vi "Populate File Info.vi"(8 "error in":errorcluster, 11 "UI Actor in":refnum<class "UI Actor.lvclass">) -> (0 "error out":errorcluster)   [LabVIEW 2019, in "UI Actor.lvlib" / "UI Actor.lvclass"]
uses:
  UI Actor.lvclass
  UI Actor.lvclass/UI Actor.ctl
  Electronic Datasheet/Electronic Datasheet.lvclass
  Core/File Info/File Info.lvclass
  Controls/File Info.ctl
  UI Actor.lvlib
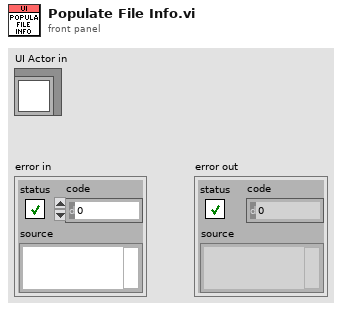
[diagram p1: front panel]
types:
  T1 = typedef "UI Actor.lvlib/File Info.ctl" = cluster{"FileVersion":u8, "FileRevision":u8, "EDSVersion":string, "Description":string, "CreationDate":string, "CreationTime":string, "CreatedBy":string, "ModificationDate":string, "ModificationTime":string, "ModifiedBy":string}
  T2 = map{path, refnum<class "Electronic Datasheet.lvclass">}
  T3 = cluster{"FileName":string, "FileVersion":u8, "FileRevision":u8, "EDSVersion":string, "Description":string, "CreationTime":string, "CreationDate":string, "CreatedBy":string, "ModificationTime":string, "ModificationDate":string, "ModifiedBy":string}
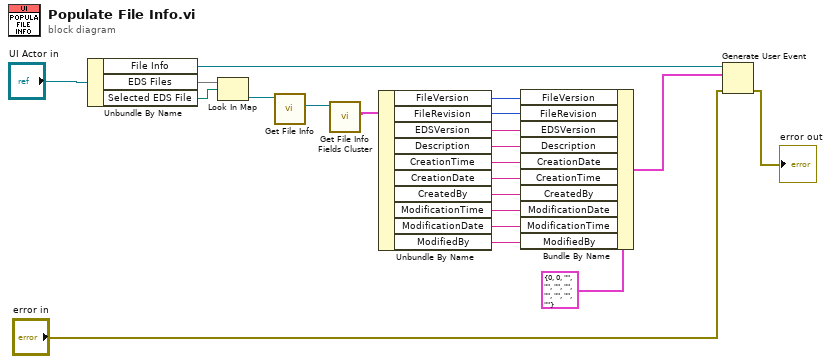
[diagram p0: block diagram]
diagram:
  n1 = Unbundle By Name("UI Actor in") -> ("File Info"=w21:refnum<user-event>, "EDS Files"=w17:T2, "Selected EDS File"=w16:path)
  n2 = Look In Map(map=w17, key=w16) -> (value=w18:refnum<class "Electronic Datasheet.lvclass">)  [unwired: 1 in, 1 out]
  n3 = call "Get File Info.vi"("reference in"=w18) -> ("File Info"=w15:refnum<class "File Info.lvclass">)  [unwired: 9 in, 1 out]
  n4 = call "Get File Info Fields Cluster.vi"("File Info in"=w15) -> ("File Info"=w14:T3)  [unwired: 9 in, 1 out]
  n5 = Unbundle By Name(w14) -> ("FileVersion"=w12:u8, "FileRevision"=w11:u8, "EDSVersion"=w10:string, "Description"=w9:string, "CreationTime"=w8:string, "CreationDate"=w7:string, "CreatedBy"=w6:string, "ModificationTime"=w5:string, "ModificationDate"=w4:string, "ModifiedBy"=w3:string)
  n6 = Bundle By Name(cluster=T1 {"FileVersion"=0, "FileRevision"=0, "EDSVersion"="", "Description"="", "CreationDate"="", "CreationTime"="", "CreatedBy"="", "ModificationDate"="", "ModificationTime"="", "ModifiedBy"=""} ("EDS File Info"), "FileVersion"=w12, "FileRevision"=w11, "EDSVersion"=w10, "Description"=w9, "CreationDate"=w8, "CreationTime"=w7, "CreatedBy"=w6, "ModificationDate"=w5, "ModificationTime"=w4, "ModifiedBy"=w3) -> (w2:T1)
  n7 = Generate User Event(user event=w21, event data cluster=w2, error in="error in") -> (error out=→"error out":errorcluster)  [unwired: 1 in, 1 out]
